vi "AtSpectrograph_logEvent_reportedDisperserPosition.vi"(8 "error in (no error)":errorcluster, 11 "logevent_reportedDisperserPosition_Ctl":T1) -> (0 "error out":errorcluster, 2 "function return":i32, 3 "logevent_reportedDisperserPosition_Ctl out":T1)   [LabVIEW 2016, in "SALLV_AtSpectrograph.lvlib"]
doc: "int AtSpectrograph_shm_logEvent_reportedDisperserPositionLV(AtSpectrograph_logevent_reportedDisperserPositionLV *logevent_reportedDisperserPosition_Ctl );"
uses:
  SALLV_AtSpectrograph.lvlib
  DataTypes/logevent_reportedDisperserPosition.ctl
  SALLV_AtSpectrograph.so
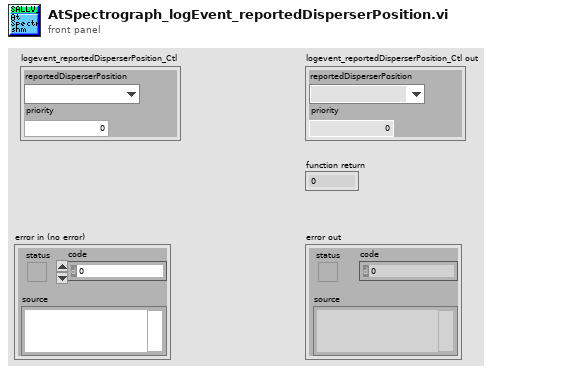
[diagram p1: front panel]
types:
  T1 = typedef "SALLV_AtSpectrograph.lvlib/logevent_reportedDisperserPosition.ctl" = cluster{"reportedDisperserPosition":enum32{"", "disperser0", "disperser1", "disperser2", "disperser3", "inbetween"}, "priority":i32}
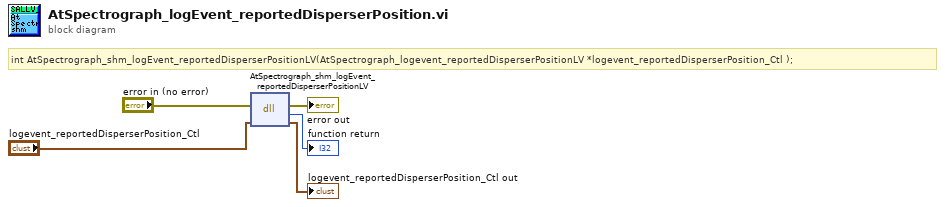
[diagram p0: block diagram]
diagram:
  # "int AtSpectrograph_shm_logEvent_reportedDisperserPositionLV(AtSpectrograph_logevent_reportedDisperserPositionLV *logevent_reportedDisperserPosition_Ctl );"
  n1 = dll-call lib="home/harini/TCS/SALLV_AtSpectrograph/SALLV_AtSpectrograph.*" fn="AtSpectrograph_shm_logEvent_reportedDisperserPositionLV"(error in="error in (no error)", "logevent_reportedDisperserPosition_Ctl"="logevent_reportedDisperserPosition_Ctl") -> (error out=→"error out":errorcluster, →"function return":i32, "logevent_reportedDisperserPosition_Ctl"=→"logevent_reportedDisperserPosition_Ctl out":T1)  [unwired: 2 in, 1 out]
